vi "TerminalConfig.vi"(11 "Args":string[](array[string])) -> (1 "Com UDP 2":T1={"UDP GrSim TX"=TRUE, "Address:"="192.168.0.101", "Port:"=20011}, 2 "RefBox UDP RX 2":T2={"Local IP:"="", "Port"=10003, "Server IP:"="224.5.23.1"}, 3 "SSL UDP RX 2":T2={"Local IP:"="192.168.0.102", "Port"=10020, "Server IP:"="224.5.23.2"}, 4 "Side 2":enum16{"Esquerdo", "Direito"}(ring) caption="Enum", 6 "Team 2":enum16{"Azul", "Amarelo"}(ring) caption="Enum")   [LabVIEW 2020]
uses:
  Controls/vision_control.ctl
  Controls/ComUDP.ctl
panel:
  out "Exit":i32
  out "Output":string
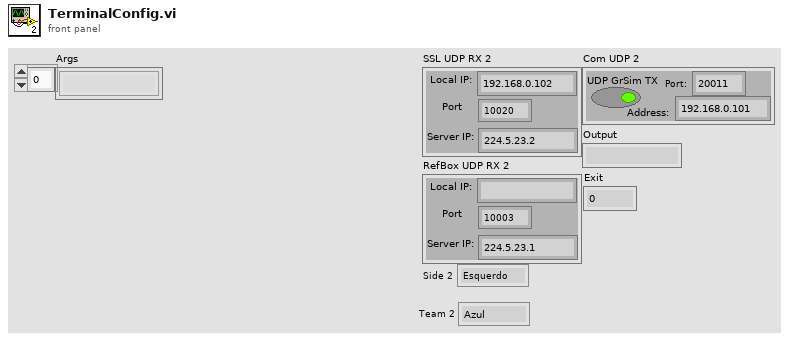
[diagram p1: front panel]
types:
  T1 = typedef "ComUDP.ctl" = cluster{"UDP GrSim TX":bool, "Address:":string, "Port:":u16}
  T2 = typedef "vision_control.ctl" = cluster{"Local IP:":string, "Port":i32, "Server IP:":string}
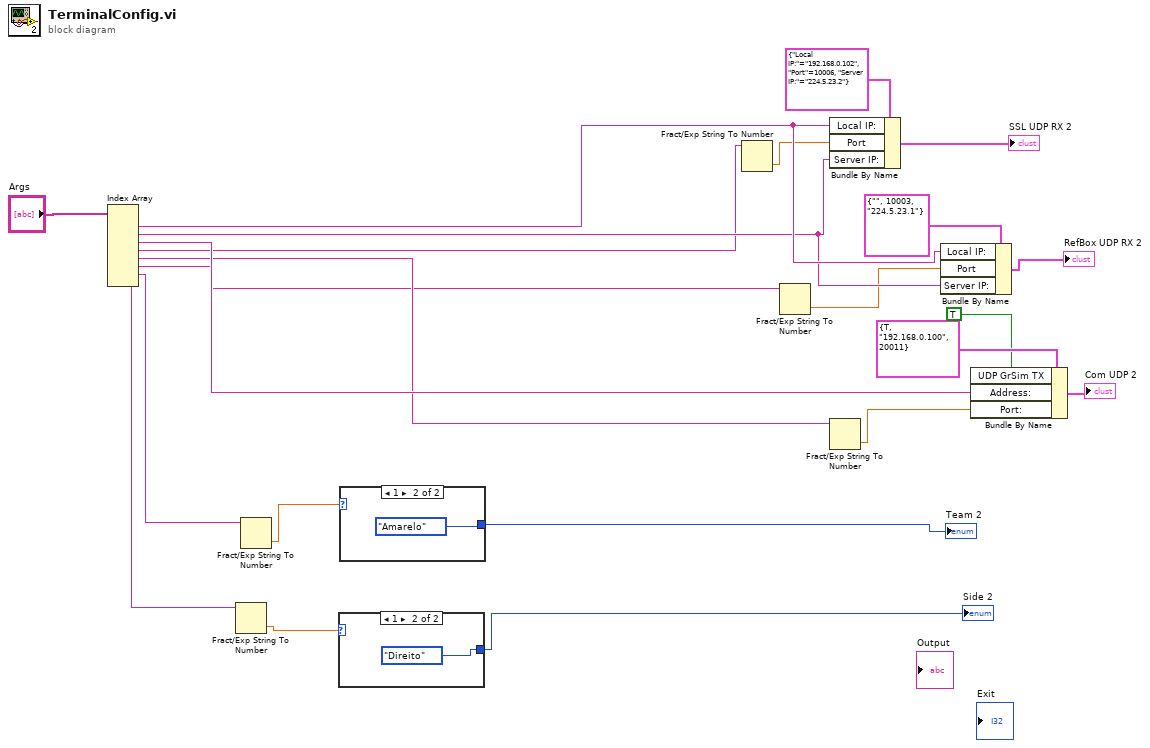
[diagram p0: block diagram]
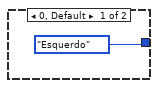
[diagram p2: hidden frame]
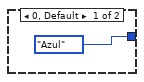
[diagram p3: hidden frame]
diagram:
  n1 = Index Array(array="Args") -> (element #1=w16:string, element #2=w15:string, element #3=w14:string, element #4=w9:string, element #5=w8:string, element #6=w7:string, element #7=w6:string, element #8=w5:string)  [unwired: 8 in]
  n2 = Fract/Exp String To Number(string=w5) -> (number=w4:dbl)  [unwired: 3 in, 1 out]
  n3 = Fract/Exp String To Number(string=w6) -> (number=w3:dbl)  [unwired: 3 in, 1 out]
  n4 = case shown="1" w4 {
    tunnel: [enum16{"Esquerdo", "Direito"}."Esquerdo" ("Side 2") enum16{"Esquerdo", "Direito"}."Direito" ("Side 2")] -> w2
    frame 0, Default {
    }
    frame 1 {
    }
  }
  "Side 2" <- w2
  n5 = case shown="1" w3 {
    tunnel: [enum16{"Azul", "Amarelo"}."Azul" ("Team 2") enum16{"Azul", "Amarelo"}."Amarelo" ("Team 2")] -> w1
    frame 0, Default {
    }
    frame 1 {
    }
  }
  "Team 2" <- w1
  n6 = Fract/Exp String To Number(string=w9) -> (number=w12:dbl)  [unwired: 3 in, 1 out]
  n7 = Fract/Exp String To Number(string=w7) -> (number=w11:dbl)  [unwired: 3 in, 1 out]
  n8 = Bundle By Name(cluster=T2 {"Local IP:"="192.168.0.102", "Port"=10006, "Server IP:"="224.5.23.2"} ("SSL UDP RX"), "Local IP:"=w16, "Port"=w12, "Server IP:"=w15) -> (→"SSL UDP RX 2":T2)
  n9 = Fract/Exp String To Number(string=w8) -> (number=w10:dbl)  [unwired: 3 in, 1 out]
  n10 = Bundle By Name(cluster=T2 {"Local IP:"="", "Port"=10003, "Server IP:"="224.5.23.1"} ("RefBox UDP RX"), "Local IP:"=w16, "Port"=w11, "Server IP:"=w15) -> (→"RefBox UDP RX 2":T2)
  n11 = Bundle By Name(cluster=T1 {"UDP GrSim TX"=TRUE, "Address:"="192.168.0.100", "Port:"=20011} ("Com UDP"), "UDP GrSim TX"=TRUE, "Address:"=w14, "Port:"=w10) -> (→"Com UDP 2":T1)
